vi "Get Properties.vi"(8 "error in (no error)":errorcluster, 11 "TTLControl in":refnum<class "TCPController.lvclass">) -> (0 "error out":errorcluster, 2 "Properties":string[](array[string]), 3 "TTLControl out":refnum<class "TCPController.lvclass">)   [LabVIEW 2020, in "TCPController.lvclass"]
uses:
  TCPController.lvclass
  D:/Development/epl-tosca/LV Source/TTL VIs/Control Classes/Base Class/TTLController.lvclass
  Base Class/TTLController.lvclass/TTLController.ctl
  Base Class/Read When.vi
  Base Class/Read Start When.vi
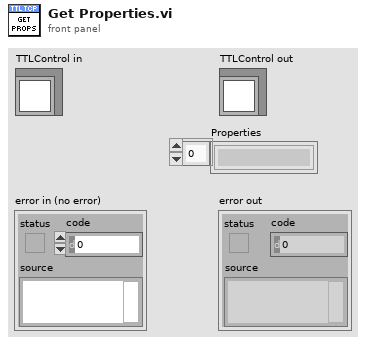
[diagram p1: front panel]
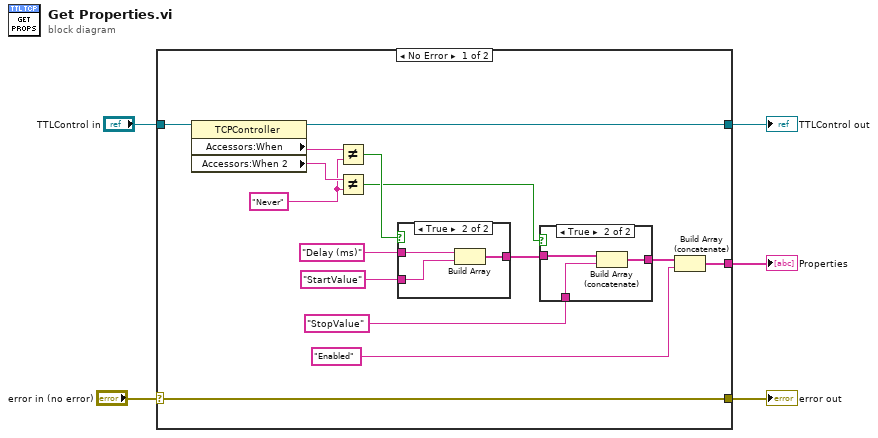
[diagram p0: block diagram]
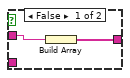
[diagram p3: hidden frame]
diagram:
  n1 = case shown="No Error" "error in (no error)" {
    selector: "error in (no error)" -> [w6 w30]
    tunnel: "TTLControl in" -> [w20 w31]
    tunnel: [w8 _] -> w4
    tunnel: [w7 w31] -> w2
    tunnel: [w6 w30] -> w1
    frame No Error {
      w16 = "Never"
      n2 = property class="TCPController"(reference=w20) -> (reference out=w7:refnum<class "TCPController.lvclass">, "Accessors:When"=w18:string, "Accessors:When 2"=w17:string)  [unwired: 1 in, 1 out]
      n3 = Not Equal?(x=w18, y=w16) -> (x != y?=w14:bool)
      n4 = Not Equal?(x=w17, y=w16) -> (x != y?=w10:bool)
      n5 = case shown="True" w14 {
        tunnel: "Delay (ms)" -> [w26 w29]
        tunnel: "StartValue" -> [_ w28]
        tunnel: [w25 w27] -> w12
        frame False {
          n6 = Build Array(w26) -> (w25:string[])
        }
        frame True {
          n7 = Build Array(w29, w28) -> (w27:string[])
        }
      }
      n8 = case shown="True" w10 {
        tunnel: w12 -> [w21 w24]
        tunnel: "StopValue" -> [_ w23]
        tunnel: [w21 w22] -> w9
        frame False {
        }
        frame True {
          n9 = Build Array (concatenate)(w24, w23) -> (w22:string[])
        }
      }
      n10 = Build Array (concatenate)(w9, "Enabled" ("element")) -> (w8:string[])
    }
    frame Error {
    }
  }
  "error out" <- w1
  "TTLControl out" <- w2
  "Properties" <- w4
